vi "crdDisplayFit_UV.vi"(9 "B":dbl, 10 "A":dbl, 11 "tau":dbl) -> (3 "Fit Out":dbl[](array[numeric]))   [LabVIEW 2011]
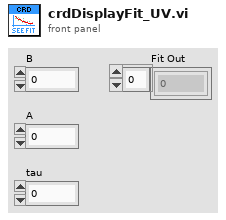
[diagram p1: front panel]
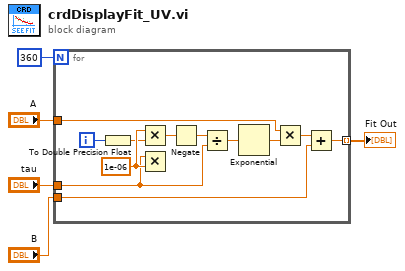
[diagram p0: block diagram]
diagram:
  n1 = for {
    N: 360 -> [_]
    tunnel: "A" -> [w17]
    tunnel: "B" -> [w11]
    tunnel: "tau" -> [w6]
    tunnel: [w10] -> w5 mode=indexing
    i -> [w8]
    w9 = 1e-06 ("x")
    n2 = To Double Precision Float(number=w8) -> (double precision float=w7:dbl)
    n3 = Multiply(x=w9, y=w7) -> (x*y=w16:dbl)
    n4 = Multiply(x=w6, y=w9) -> ()  [unwired: 1 out]
    n5 = Negate(x=w16) -> (-x=w15:dbl)
    n6 = Divide(x=w15, y=w6) -> (x/y=w14:dbl)
    n7 = Exponential(1:w14) -> (0:w13:dbl)
    n8 = Multiply(x=w17, y=w13) -> (x*y=w12:dbl)
    n9 = Add(x=w12, y=w11) -> (x+y=w10:dbl)
  }
  "Fit Out" <- w5
